vi "Data Average Plot.vi"(7 "No of element":dbl, 8 "Average file path":path, 9 "Current file path":path) -> (1 "XY Graph":cluster{"Y":dbl[], "Y":dbl[]}[](graph), 2 "Y Out":dbl[](array[numeric]), 3 "X Out":dbl[](array[numeric]))   [LabVIEW 2011]
uses:
  <vilib>/Utility/file.llb/Read From Spreadsheet File (DBL).vi
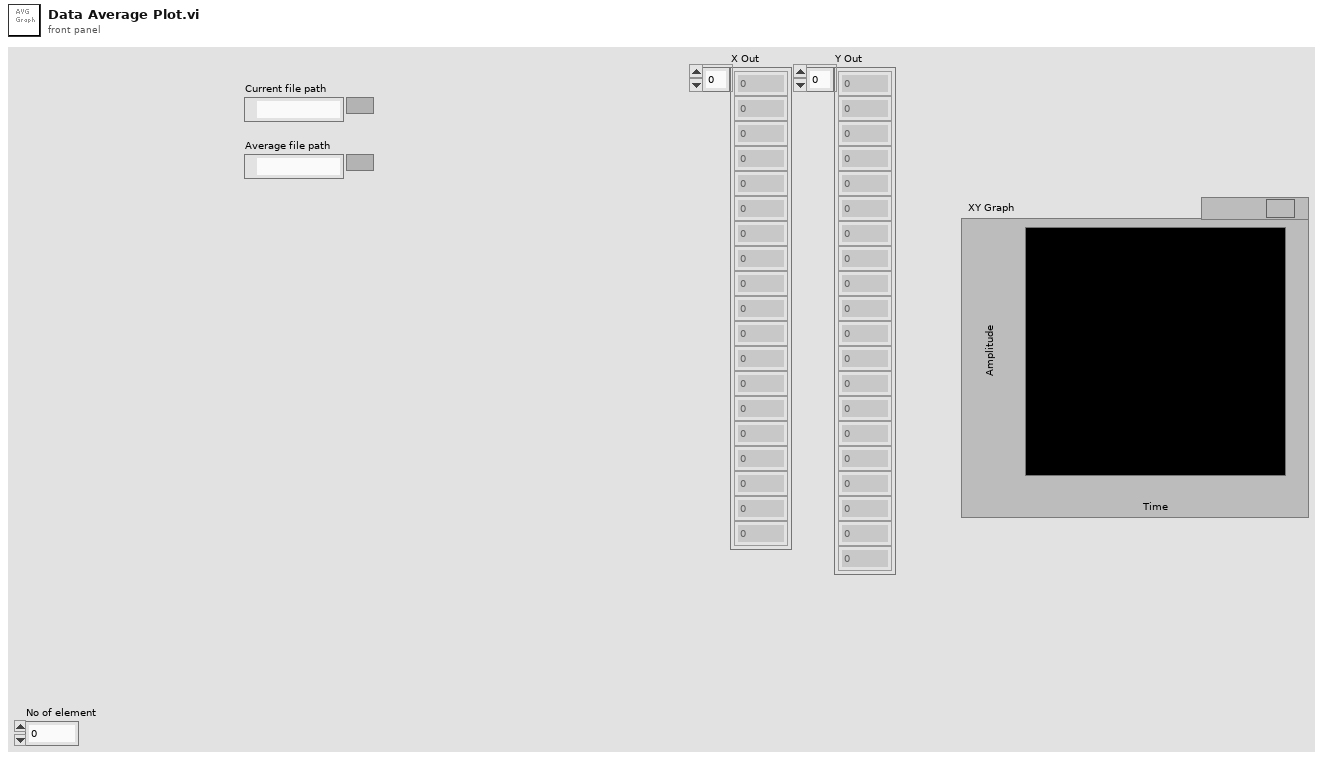
[diagram p1: front panel]
types:
  T1 = typedef "NI_Matrix.lvlib/RealMatrix.ctl" = dbl[][]
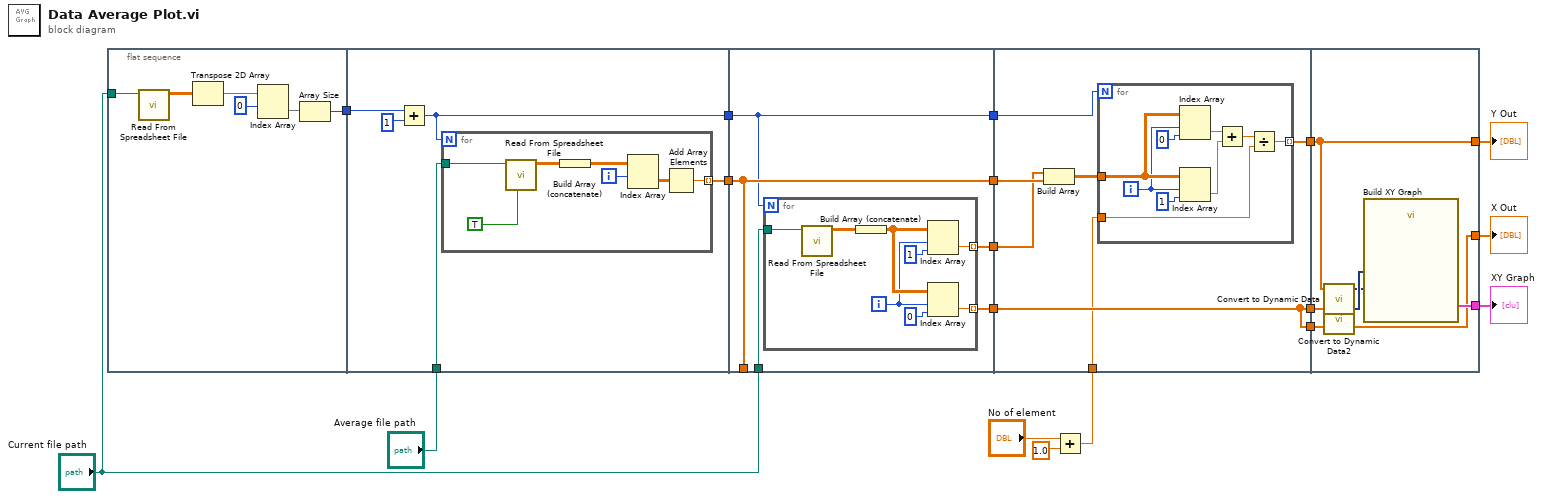
[diagram p0: block diagram]
diagram:
  n1 = flat-sequence {
    tunnel: "Current file path" -> [w20]
    tunnel: [w19] -> w14
    tunnel: [w25] -> w18
    tunnel: "Average file path" -> [w29]
    tunnel: w14 -> [w27]
    tunnel: [w26] -> w13
    tunnel: w18 -> [w38]
    tunnel: "Current file path" -> [w41]
    tunnel: w13 -> [w37]
    tunnel: [w40] -> w9
    tunnel: [w38] -> w8
    tunnel: [w39] -> w7
    tunnel: [w38] -> _
    tunnel: [w37] -> w6
    tunnel: [w56] -> w11
    tunnel: [w56] -> w10
    tunnel: w9 -> [w56]
    tunnel: w8 -> [w55]
    tunnel: w7 -> [w53]
    tunnel: w6 -> [w54]
    tunnel: w3 -> [w51]
    tunnel: [w50] -> w2
    tunnel: w11 -> [w71]
    tunnel: [w70] -> w16
    tunnel: [w67] -> w12
    tunnel: w10 -> [w67]
    tunnel: w2 -> [w66]
    tunnel: [w66] -> w1
    frame #0 {
      n2 = call-poly <vilib>:"Read From Spreadsheet File.vi"("file path (dialog if empty)"=w20) -> ("all rows"=w23:dbl[][])  [unwired: 6 in, 4 out]
      n3 = Transpose 2D Array(2D array=w23) -> (transposed array=w24:dbl[][])
      n4 = Index Array(array=w24, index (row)=0) -> (element=w22:dbl[])  [unwired: 1 in]
      n5 = Array Size(array=w22) -> (size(s)=w19:i32)
    }
    frame #1 {
      n6 = Add(x=w27, y=1) -> (x+y=w26:i32)
      n7 = for {
        N: w26 -> [_]
        tunnel: [w30] -> w25 mode=indexing
        tunnel: w29 -> [w32]
        i -> [w34]
        n8 = call-poly <vilib>:"Read From Spreadsheet File.vi"("transpose (no:F)"=TRUE, "file path (dialog if empty)"=w32) -> ("all rows"=w35:dbl[][])  [unwired: 5 in, 4 out]
        n9 = Build Array (concatenate)(w35) -> (w33:T1)
        n10 = Index Array(array=w33, index (row)=w34) -> (element=w31:T1)  [unwired: 1 in]
        n11 = Add Array Elements(numeric array=w31) -> (sum=w30:dbl)
      }
    }
    frame #2 {
      n12 = for {
        N: w37 -> [_]
        tunnel: [w48] -> w40 mode=indexing
        tunnel: w41 -> [w46]
        tunnel: [w44] -> w39 mode=indexing
        i -> [w42]
        n13 = call-poly <vilib>:"Read From Spreadsheet File.vi"("file path (dialog if empty)"=w46) -> ("all rows"=w49:dbl[][])  [unwired: 6 in, 4 out]
        n14 = Build Array (concatenate)(w49) -> (w45:T1)
        n15 = Index Array(array=w45, index (row)=w42, index (col)=1 ("index (row)")) -> (element=w44:dbl)
        n16 = Index Array(array=w45, index (row)=w42, index (col)=0) -> (element=w48:dbl)
      }
    }
    frame #3 {
      n17 = Build Array(w53, w55) -> (w52:T1)
      n18 = for {
        N: w54 -> [_]
        tunnel: w52 -> [w64]
        tunnel: [w57] -> w50 mode=indexing
        tunnel: w51 -> [w58]
        i -> [w62]
        n19 = Index Array(array=w64, index (row)=w62, index (col)=0) -> (element=w61:dbl)
        n20 = Index Array(array=w64, index (row)=w62, index (col)=1) -> (element=w60:dbl)
        n21 = Add(x=w61, y=w60) -> (x+y=w59:dbl)
        n22 = Divide(x=w59, y=w58) -> (x/y=w57:dbl)
      }
    }
    frame #4 {
      n23 = call "Convert to Dynamic Data"("Array"=w66) -> ("Dynamic Data Type"=w68:dynamicdata)  [unwired: 3 in]
      n24 = call "Convert to Dynamic Data2"("Array"=w71) -> ("Dynamic Data Type"=w69:dynamicdata)  [unwired: 3 in]
      n25 = call "Build XY Graph"("Y Input"=w68, "X Input"=w69) -> ("XY Graph"=w70:cluster{"Y":dbl[], "Y":dbl[]}[])  [unwired: 3 in, 6 out]
    }
  }
  n26 = Add(x="No of element", y=1.0) -> (x+y=w3:dbl)
  "XY Graph" <- w16
  "X Out" <- w12
  "Y Out" <- w1
